vi "Actor Core.vi"(8 "error in":errorcluster, 11 "Create Sensor View in":refnum<class "Create Sensor View.lvclass">) -> (0 "error out":errorcluster, 3 "Actor out":refnum<class "Actor.lvclass">)   [LabVIEW 2013, in "Create Sensor View.lvlib" / "Create Sensor View.lvclass"]
doc: "(<B>Filename</B>: Actor Framework.lvlib:Actor.lvclass:Actor Core.vi)\n\nReceives messages to the actor, reacts to them, and initiates any error handling that may shut the actor down.\n\nDescendant classes may override this VI to append parallel tasks for the actor to complete while it handles messages. Overrides use the Call Parent Method node."
uses:
  Create Sensor View.lvclass
  <vilib>/ActorFramework/Actor/Actor.lvclass
  Resources/UI Controls/Common/Side Button.ctl
  <vilib>/ActorFramework/Actor/Actor.lvclass/Actor.ctl
  <vilib>/ActorFrameworkMVC/View Actor/View Actor.lvclass
  <vilib>/ActorFramework/Message Enqueuer/Message Enqueuer.lvclass/Message Enqueuer.ctl
  Create Sensor View.lvclass/Create Sensor View.ctl
  <vilib>/Utility/miscctls.llb/LVPositionTypeDef.ctl
  <vilib>/ActorFrameworkMVC/UI Controller Messages/Move Subpanel Msg/Move Subpanel Msg.lvclass/Move Subpanel Msg.ctl
  <vilib>/ActorFrameworkMVC/UI Controller Messages/Insert Subpanel Msg/Insert Subpanel Msg.lvclass/Insert Subpanel Msg.ctl
  Models/Create Sensor Model Messages/Set Item Configurations Msg/Set Item Configurations Msg.lvclass/Set Item Configurations Msg.ctl
  <vilib>/ActorFramework/Message Enqueuer/Init from Existing Queue.vi
  <vilib>/ActorFramework/Message Enqueuer/Enqueue.vi
  <vilib>/ActorFramework/Message Priority Queue/Priority Enqueue.vi
  <vilib>/ActorFramework/Message Enqueuer/Message Enqueuer.lvclass
  <vilib>/ActorFrameworkMVC/UI Controller Messages/Move Subpanel Msg/Move Subpanel Msg.lvclass
  <vilib>/ActorFrameworkMVC/UI Controller Messages/Insert Subpanel Msg/Insert Subpanel Msg.lvclass
  Models/Create Sensor Model Messages/Set Item Configurations Msg/Set Item Configurations Msg.lvclass
  Models/Create Sensor Model Messages/Create Sensor Msg/Create Sensor Msg.lvclass
  Models/Sensor Model Messages/Preview Sensor Msg/Preview Sensor Msg.lvclass
  Models/Sensor Model Messages/Update Tiles Info Msg/Update Tiles Info Msg.lvclass
  Models/Sensor Model Messages/Update Previous Button Visibility Msg/Update Previous Button Visibility Msg.lvclass
  Models/Sensor Model Messages/Update Next Button Visibility Msg/Update Next Button Visibility Msg.lvclass
  Common/File IO/File IO.lvlib
  <vilib>/ActorFrameworkMVC/UI Controller Messages/Get Model Actor Enqueuer Msg/Get Model Actor Enqueuer Msg.lvclass
  <vilib>/ActorFrameworkMVC/View Actor Messages/Get Model Enqueuer Msg/Get Model Enqueuer Msg.lvclass
  Resources/UI Controls/UI Control.lvlib
panel:
  in  "Cancel":bool
  in  "Save":bool
  out "Tab Control":enum32{"Basic Info"}(tab)
  in  "Sensor Unit":string caption="传感器单位："
  in  "HR":string caption="传感器实际量程（HR）："
  in  "LR":string caption="传感器实际量程（LR）："
  in  "HV":string caption="传感器电压范围（HV）："
  in  "Sensor Description":string caption="传感器描述："
  in  "Sensor Name":string caption="传感器名称："
  in  "LV":string caption="传感器电压范围（LV）："
  in  "Side Buttons":enum32{"Basic Info"}(radio)
  # "新建传感器"
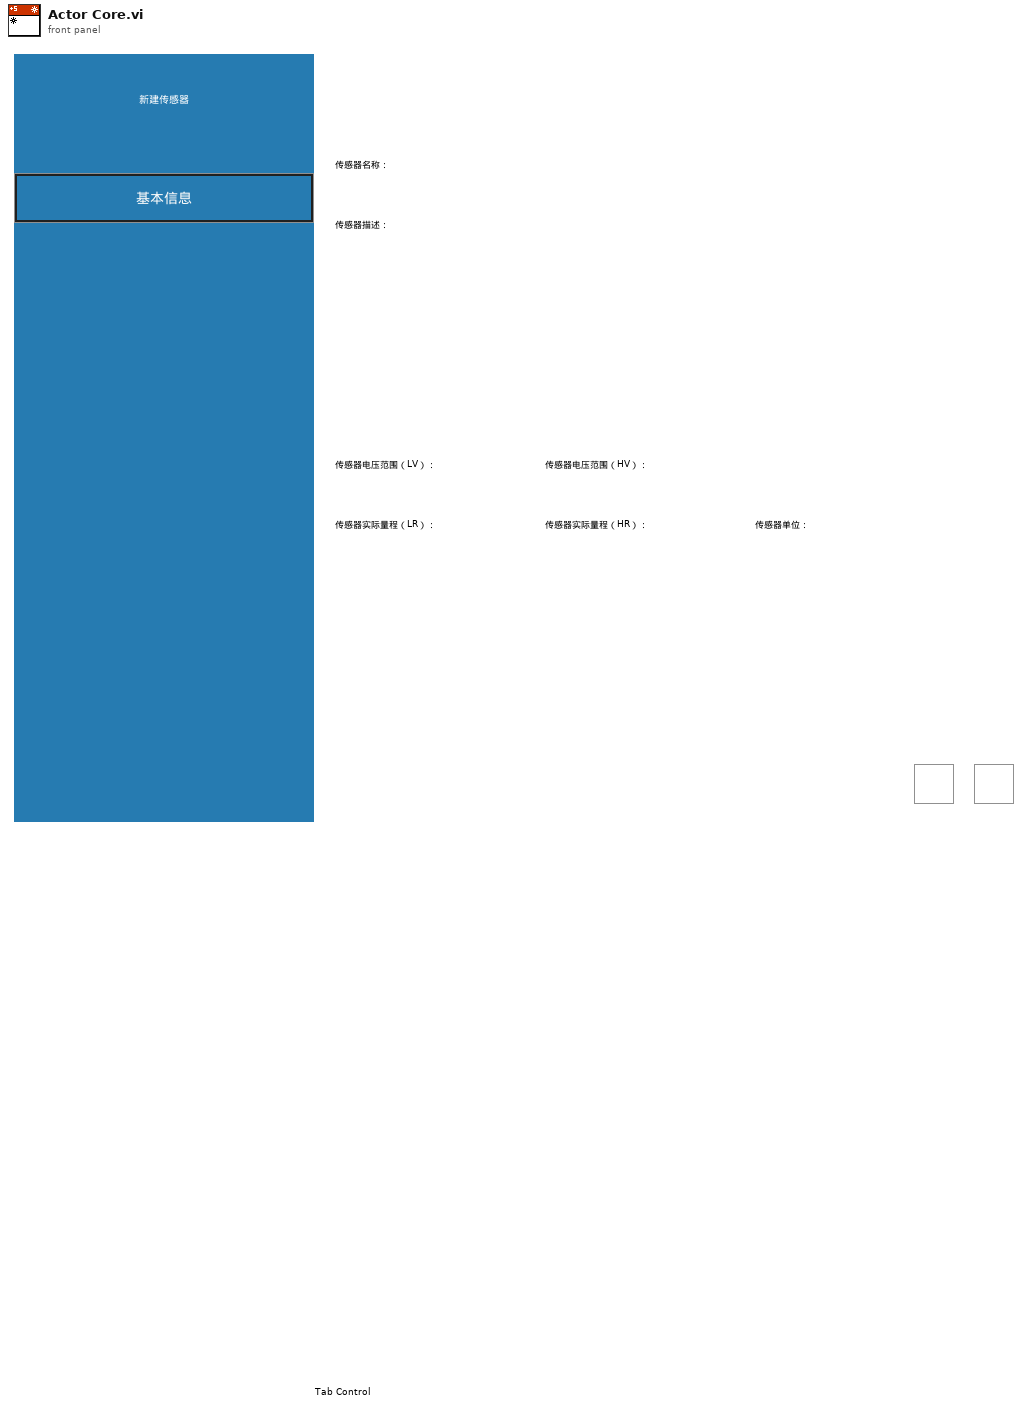
[diagram p1: front panel]
types:
  T1 = typedef "Create Sensor View.lvlib/Create Sensor View.lvclass/Events.ctl" = cluster{"Reinitialize All":refnum<user-event>, "Key Focus":refnum<user-event>}
  T2 = typedef "LVPositionTypeDef.ctl" = cluster{"Left":i32, "Top":i32}
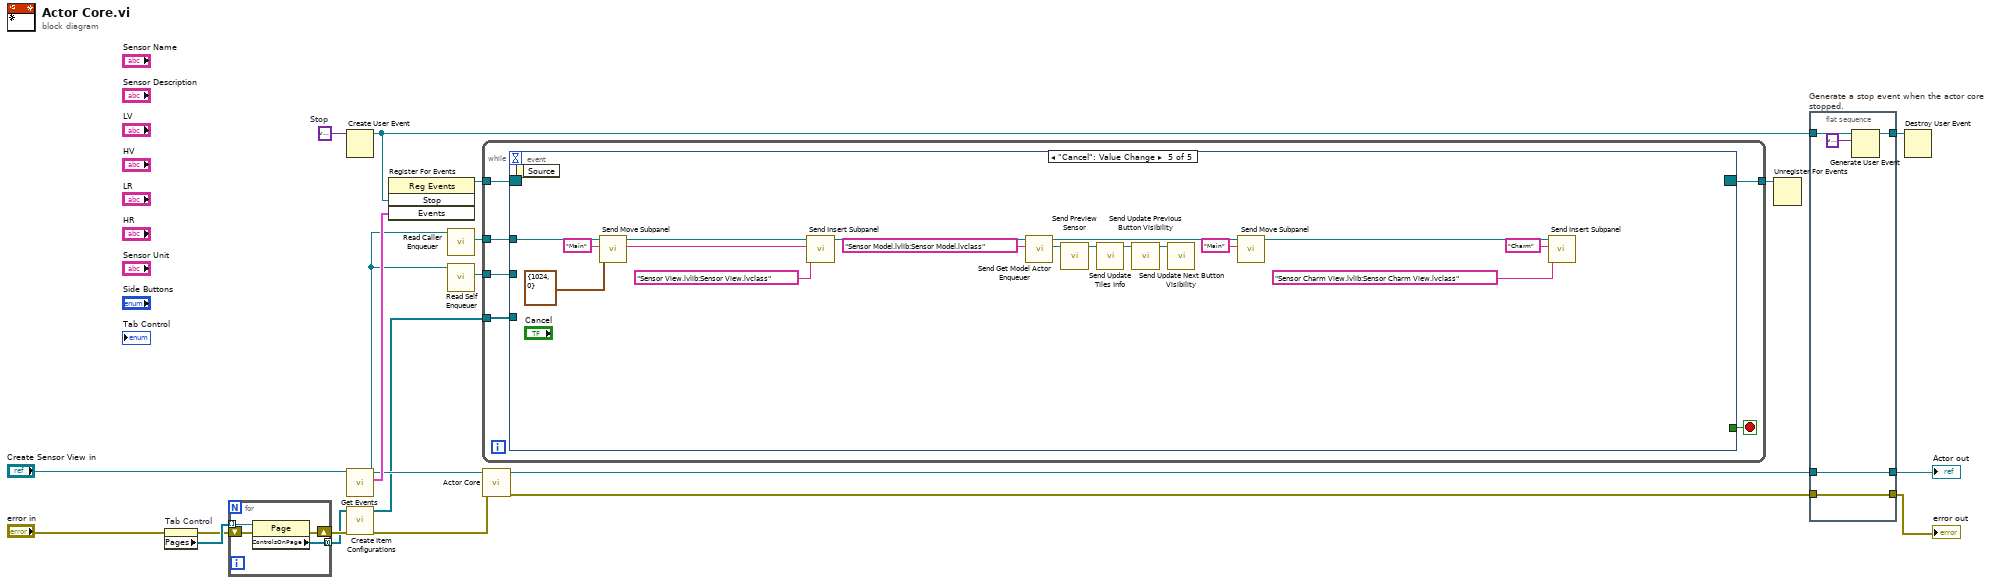
[diagram p0: block diagram]
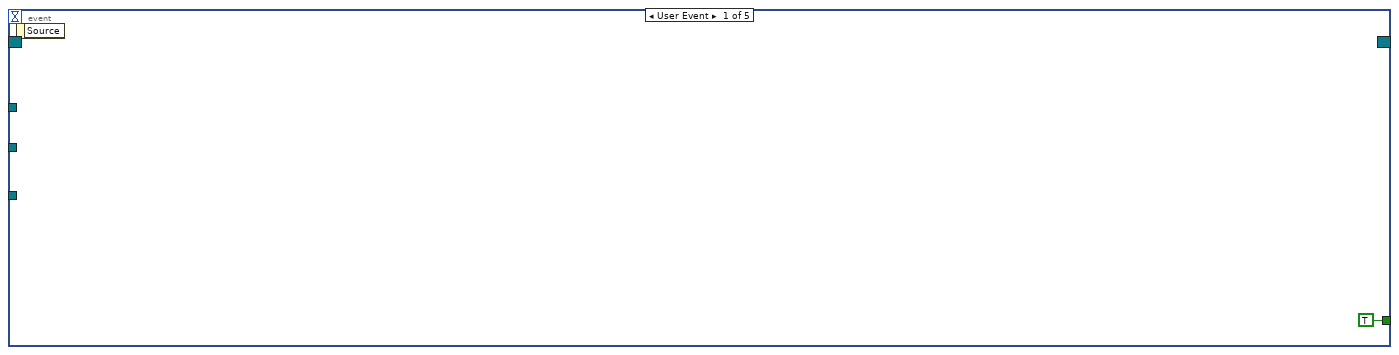
[diagram p2: hidden frame]
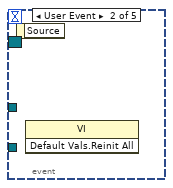
[diagram p3: hidden frame]
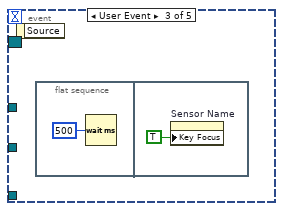
[diagram p4: hidden frame]
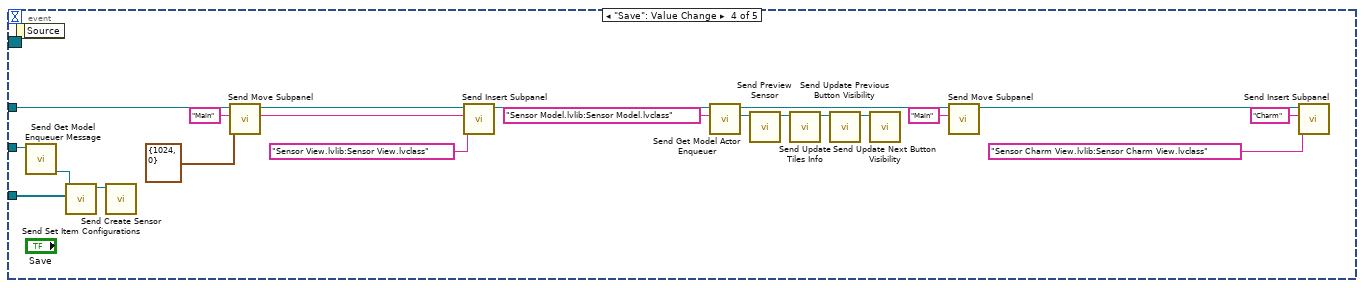
[diagram p5: hidden frame]
diagram:
  w21 = variant  # Stop
  n1 = property on="Tab Control" class="TabCtl (strict)"(error in="error in") -> (error out=w9:errorcluster, "Pages"=w10:refnum<vi>[])  [unwired: 1 in, 1 out]
  n2 = for {
    tunnel: w10 -> [w25] mode=indexing
    tunnel: [w24] -> w7 mode=concatenating
    shift-right: [w22] -> w8
    shift-left: w9 -> [w23]
    n3 = property class="Page"(reference=w25, error in=w23) -> (error out=w22:errorcluster, "ControlsOnPage"=w24:refnum<vi>[])  [unwired: 1 out]
  }
  n4 = Create User Event(user event datatype=w21) -> (user event=w13:refnum<user-event>)  [unwired: 1 in, 1 out]
  n5 = call "Get Events.vi"("Create Sensor View in"="Create Sensor View in") -> ("Events"=w12:T1, "Create Sensor View out"=w2:refnum<class "Create Sensor View.lvclass">)  [unwired: 9 in]
  n6 = call "Create Item Configurations.vi"("error in (no error)"=w8, "Controls References"=w7) -> ("error out"=w5:errorcluster, "Item Configurations"=w1:refnum<class "Item Configuration.lvclass">[])  [unwired: 8 in]
  n7 = register-events(w13, w12) -> (reference out=w14:refnum<event-registration>)  [unwired: 2 in, 1 out]
  n8 = call <vilib>:"Read Caller Enqueuer.vi"("Actor"=w2) -> ("Caller Enqueuer"=w4:refnum<class "Message Enqueuer.lvclass">)  [unwired: 10 in]
  n9 = call <vilib>:"Read Self Enqueuer.vi"("Actor"=w2) -> ("Self Enqueuer"=w3:refnum<class "Message Enqueuer.lvclass">)  [unwired: 10 in]
  n10 = while {
    tunnel: [w31] -> w11
    tunnel: w14 -> [w29]
    tunnel: w4 -> [w28]
    tunnel: w3 -> [w27]
    tunnel: w1 -> [w26]
    stop <- w30 stop-if-true
    n11 = event shown="[4] \"Cancel\": Value Change" {
      selector: w29 -> [_ _ _ _ _]
      dyn-events: [_ _ _ _ _] -> w31
      timeout: _ -> [_ _ _ _ _]
      tunnel: [TRUE _ _ _ _] -> w30
      tunnel: w28 -> [_ _ _ w40 w56]
      tunnel: w27 -> [_ _ _ w36 _]
      tunnel: w26 -> [_ _ _ w35 _]
      event User Event {
        n12 = event-data() -> ()  [unwired: 1 in, 1 out]
      }
      event User Event {
        n13 = event-data() -> ()  [unwired: 1 in, 1 out]
        n14 = invoke class="VI" method="Default Vals.Reinit All"() -> ()  [unwired: 3 in, 3 out]
      }
      event User Event {
        n15 = event-data() -> ()  [unwired: 1 in, 1 out]
        n16 = flat-sequence {
          frame #0 {
            n17 = Wait (ms)(milliseconds to wait=u32 500) -> ()  [unwired: 1 out]
          }
          frame #1 {
            n18 = property on="Sensor Name" class="Str"("Key Focus"=TRUE) -> ()  [unwired: 2 in, 2 out]
          }
        }
      }
      event "Save": Value Change {
        w51 = "Main" ("Subpanel Name")
        n19 = event-data() -> ()  [unwired: 1 in, 1 out]
        n20 = call <vilib>:"Send Get Model Enqueuer Message.vi"("Message Enqueuer in"=w36) -> ("Reply"=w38:refnum<class "Message Enqueuer.lvclass">)  [unwired: 7 in, 3 out]
        n21 = call "Send Set Item Configurations.vi"("Item Configurations"=w35, "Message Enqueuer"=w38) -> ("Message Enqueuer out"=w37:refnum<class "Message Enqueuer.lvclass">)  [unwired: 8 in, 1 out]
        n22 = call "Send Create Sensor.vi"("Message Enqueuer"=w37) -> ()  [unwired: 9 in, 2 out]
        n23 = call <vilib>:"Send Move Subpanel.vi"("Position (0,0)"=T2 {"Left"=1024, "Top"=0}, "Subpanel Name"=w51, "Message Enqueuer"=w40) -> ("Message Enqueuer out"=w54:refnum<class "Message Enqueuer.lvclass">)  [unwired: 7 in, 1 out]
        n24 = call <vilib>:"Send Insert Subpanel.vi"("View Name"="Sensor View.lvlib:Sensor View.lvclass" ("Subpanel Name"), "Subpanel Name"=w51, "Message Enqueuer"=w54) -> ("Message Enqueuer out"=w49:refnum<class "Message Enqueuer.lvclass">)  [unwired: 7 in, 1 out]
        n25 = call <vilib>:"Send Get Model Actor Enqueuer.vi"("Model Name"="Sensor Model.lvlib:Sensor Model.lvclass", "Message Enqueuer in"=w49) -> ("Reply"=w39:refnum<class "Message Enqueuer.lvclass">, "Message Enqueuer out"=w48:refnum<class "Message Enqueuer.lvclass">)  [unwired: 6 in, 2 out]
        n26 = call "Send Preview Sensor.vi"("Message Enqueuer"=w39) -> ("Message Enqueuer out"=w45:refnum<class "Message Enqueuer.lvclass">)  [unwired: 9 in, 1 out]
        n27 = call "Send Update Tiles Info.vi"("Message Enqueuer"=w45) -> ("Message Enqueuer out"=w44:refnum<class "Message Enqueuer.lvclass">)  [unwired: 9 in, 1 out]
        n28 = call "Send Update Previous Button Visibility.vi"("Message Enqueuer"=w44) -> ("Message Enqueuer out"=w43:refnum<class "Message Enqueuer.lvclass">)  [unwired: 9 in, 1 out]
        n29 = call "Send Update Next Button Visibility.vi"("Message Enqueuer"=w43) -> ()  [unwired: 9 in, 2 out]
        n30 = call <vilib>:"Send Move Subpanel.vi"("Subpanel Name"="Main", "Message Enqueuer"=w48) -> ("Message Enqueuer out"=w46:refnum<class "Message Enqueuer.lvclass">)  [unwired: 8 in, 1 out]
        n31 = call <vilib>:"Send Insert Subpanel.vi"("View Name"="Sensor Charm View.lvlib:Sensor Charm View.lvclass", "Subpanel Name"="Charm", "Message Enqueuer"=w46) -> ()  [unwired: 7 in, 2 out]
      }
      event "Cancel": Value Change {
        w67 = "Main" ("Subpanel Name")
        n32 = event-data() -> ()  [unwired: 1 in, 1 out]
        n33 = call <vilib>:"Send Move Subpanel.vi"("Position (0,0)"=T2 {"Left"=1024, "Top"=0}, "Subpanel Name"=w67, "Message Enqueuer"=w56) -> ("Message Enqueuer out"=w70:refnum<class "Message Enqueuer.lvclass">)  [unwired: 7 in, 1 out]
        n34 = call <vilib>:"Send Insert Subpanel.vi"("View Name"="Sensor View.lvlib:Sensor View.lvclass" ("Subpanel Name"), "Subpanel Name"=w67, "Message Enqueuer"=w70) -> ("Message Enqueuer out"=w65:refnum<class "Message Enqueuer.lvclass">)  [unwired: 7 in, 1 out]
        n35 = call <vilib>:"Send Get Model Actor Enqueuer.vi"("Model Name"="Sensor Model.lvlib:Sensor Model.lvclass", "Message Enqueuer in"=w65) -> ("Reply"=w55:refnum<class "Message Enqueuer.lvclass">, "Message Enqueuer out"=w64:refnum<class "Message Enqueuer.lvclass">)  [unwired: 6 in, 2 out]
        n36 = call "Send Preview Sensor.vi"("Message Enqueuer"=w55) -> ("Message Enqueuer out"=w61:refnum<class "Message Enqueuer.lvclass">)  [unwired: 9 in, 1 out]
        n37 = call "Send Update Tiles Info.vi"("Message Enqueuer"=w61) -> ("Message Enqueuer out"=w60:refnum<class "Message Enqueuer.lvclass">)  [unwired: 9 in, 1 out]
        n38 = call "Send Update Previous Button Visibility.vi"("Message Enqueuer"=w60) -> ("Message Enqueuer out"=w59:refnum<class "Message Enqueuer.lvclass">)  [unwired: 9 in, 1 out]
        n39 = call "Send Update Next Button Visibility.vi"("Message Enqueuer"=w59) -> ()  [unwired: 9 in, 2 out]
        n40 = call <vilib>:"Send Move Subpanel.vi"("Subpanel Name"="Main", "Message Enqueuer"=w64) -> ("Message Enqueuer out"=w62:refnum<class "Message Enqueuer.lvclass">)  [unwired: 8 in, 1 out]
        n41 = call <vilib>:"Send Insert Subpanel.vi"("View Name"="Sensor Charm View.lvlib:Sensor Charm View.lvclass", "Subpanel Name"="Charm", "Message Enqueuer"=w62) -> ()  [unwired: 7 in, 2 out]
      }
    }
  }
  n42 = call-parent "Actor Core.vi"("error in"=w5, "View Actor in"=w2) -> ("error out"=w17:errorcluster, "Actor out"=w18:refnum<class "Actor.lvclass">)  [unwired: 8 in]
  n43 = Unregister For Events(event registration refnum=w11) -> ()  [unwired: 1 in, 1 out]
  n44 = flat-sequence "Generate a stop event when the actor core stopped." {
    tunnel: w13 -> [w75]
    tunnel: [w73] -> w20
    tunnel: w18 -> [w72]
    tunnel: w17 -> [w71]
    tunnel: [w72] -> w16
    tunnel: [w71] -> w15
    frame #0 {
      n45 = Generate User Event(user event=w75, event data cluster=variant ("event data")) -> (user event out=w73:refnum<user-event>)  [unwired: 2 in, 1 out]
    }
  }
  n46 = Destroy User Event(user event=w20) -> ()  [unwired: 1 in, 1 out]
  "error out" <- w15
  "Actor out" <- w16
